vi "InitADCHannel.vi"(1 "error out":errorcluster) -> (0 "Boolean":bool, 2 "number":i32, 3 "DLL error code":u32, 4 "String":string, 5 "error out 2":errorcluster)   [LabVIEW 2011]
uses:
  Variables/GlobalCameraHandle.vi
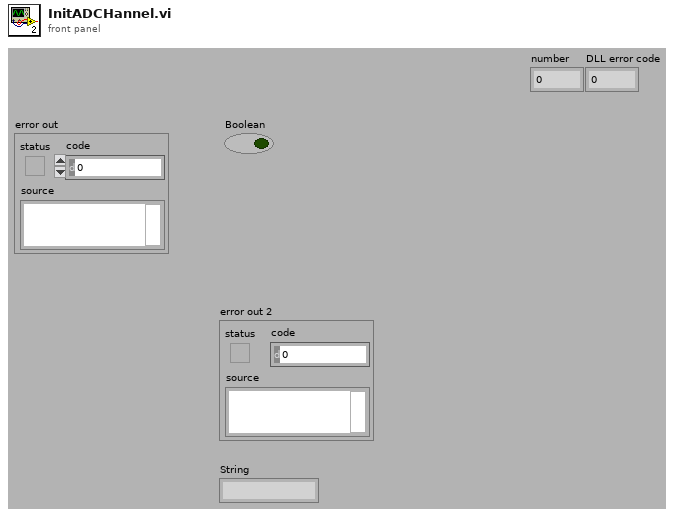
[diagram p1: front panel]
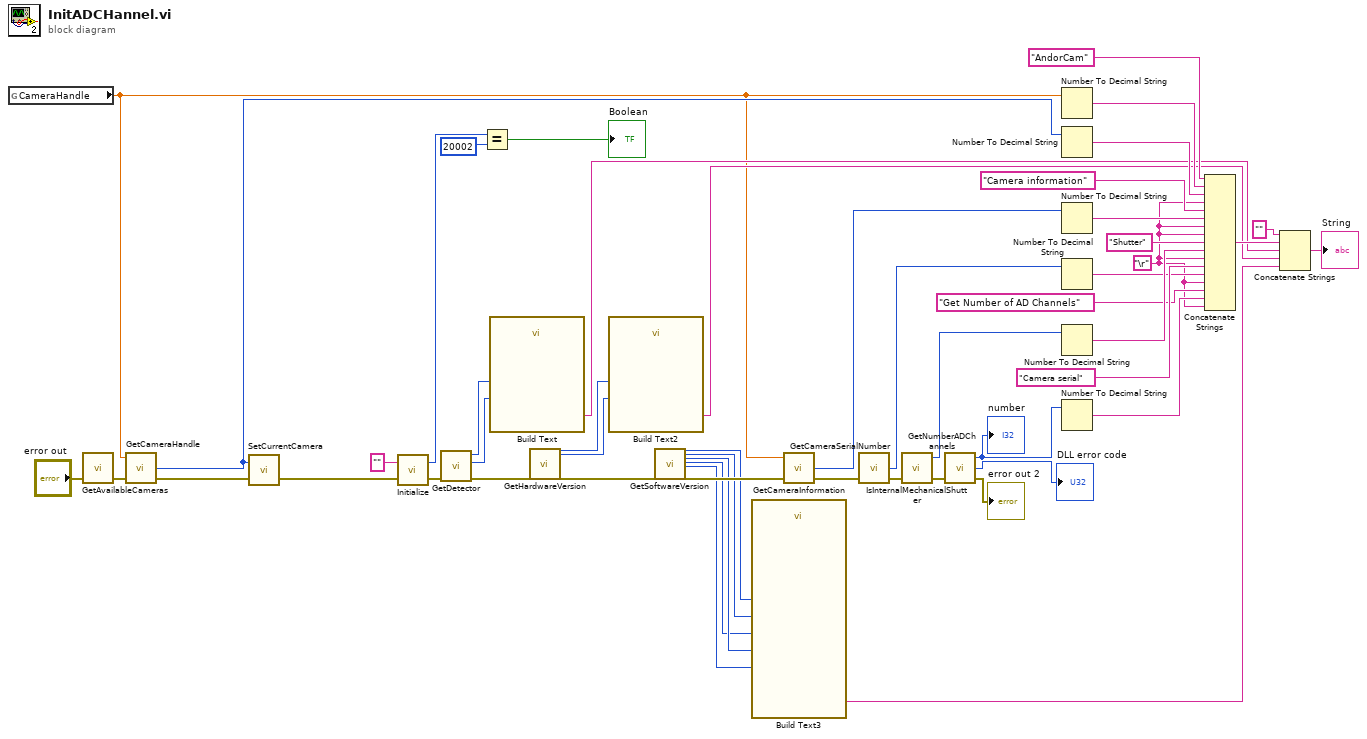
[diagram p0: block diagram]
diagram:
  w11 = "\r"
  n1 = global read "GlobalCameraHandle.vi" "CameraHandle"() -> (w1:dbl)
  n2 = call "GetAvailableCameras.vi"("error in (no error)"="error out") -> ("error out"=w49:errorcluster)  [unwired: 2 in, 2 out]
  n3 = call "GetCameraHandle.vi"("error in (no error)"=w49, "cameraIndex"=w1) -> ("error out"=w40:errorcluster, "cameraHandle"=w3:i32)  [unwired: 1 in, 1 out]
  n4 = call "SetCurrentCamera.vi"("error in (no error)"=w40, "cameraHandle"=w3) -> ("error out"=w39:errorcluster)  [unwired: 1 out]
  n5 = call "Initialize.vi"("error in (no error)"=w39, "directory (\"\")"="" ("directory (\"\")")) -> ("error out"=w41:errorcluster, "DLL error code"=w10:u32)
  n6 = call "GetDetector.vi"("error in (no error)"=w41) -> ("error out"=w42:errorcluster, "ypixels"=w31:i32, "xpixels"=w32:i32)  [unwired: 3 in, 1 out]
  n7 = Equal?(x=w10, y=u32 20002) -> (x = y?=→"Boolean":bool)
  n8 = call "Build Text"("x"=w32, "y"=w31) -> ("Result"=w8:string)  [unwired: 12 in, 1 out]
  n9 = call "GetHardwareVersion.vi"("error in (no error)"=w42) -> ("PCB"=w30:u32, "Flex"=w29:u32, "error out"=w38:errorcluster)  [unwired: 19 in, 5 out]
  n10 = call "Build Text2"("pcb"=w30, "FLEX"=w29) -> ("Result"=w7:string)  [unwired: 12 in, 1 out]
  n11 = call "GetSoftwareVersion.vi"("error in (no error)"=w38) -> ("eprom"=w28:u32, "cofFile"=w27:u32, "vxdRev"=w26:u32, "vxdVer"=w25:u32, "dllRev"=w24:u32, "error out"=w43:errorcluster)  [unwired: 19 in, 2 out]
  n12 = call "Build Text3"("vxdrew"=w26, "eprom"=w28, "con"=w27, "vxdver"=w25, "dllrev"=w24) -> ("Result"=w6:string)  [unwired: 9 in, 1 out]
  n13 = call "GetCameraInformation.vi"("error in (no error)"=w43, "index"=w1) -> ("error out"=w37:errorcluster, "information"=w21:i32)  [unwired: 1 in, 1 out]
  n14 = call "GetCameraSerialNumber.vi"("error in (no error)"=w37) -> ("error out"=w4:errorcluster, "number"=w15:i32)  [unwired: 2 in, 1 out]
  n15 = call "IsInternalMechanicalShutter.vi"("error in (no error)"=w4) -> ("error out"=w46:errorcluster, "DLL error code"=w18:u32)  [unwired: 2 in, 1 out]
  n16 = call "GetNumberADChannels.vi"("error in (no error)"=w46) -> ("error out"=→"error out 2":errorcluster, "DLL error code"=→"DLL error code":u32, "number"=w13:i32)  [unwired: 2 in]
  "number" <- w13
  n17 = Number To Decimal String(number=w1) -> (decimal integer string=w45:string)  [unwired: 1 in]
  n18 = Number To Decimal String(number=w3) -> (decimal integer string=w33:string)  [unwired: 1 in]
  n19 = Number To Decimal String(number=w21) -> (decimal integer string=w22:string)  [unwired: 1 in]
  n20 = Number To Decimal String(number=w15) -> (decimal integer string=w16:string)  [unwired: 1 in]
  n21 = Number To Decimal String(number=w18) -> (decimal integer string=w19:string)  [unwired: 1 in]
  n22 = Number To Decimal String(number=w13) -> (decimal integer string=w12:string)  [unwired: 1 in]
  n23 = Concatenate Strings("AndorCam" ("directory (\"\")"), w45, w33, w11, "Camera information" ("string"), w22, w11, w11, "Shutter" ("string"), w19, w11, "Camera serial" ("string"), w16, w11, "Get Number of AD Channels" ("string"), w12, w11) -> (w9:string)
  n24 = Concatenate Strings("", w9, w8, w7, w6) -> (→"String":string)
